vi "Set DDG External Output Enabled.vi"(8 "error in (no error)":errorcluster, 10 "uiEnabled":u32, 11 "uiIndex":u32) -> (0 "error out":errorcluster, 3 "function return":u32)   [LabVIEW 2014, in "atmcd32d.lvlib"]
doc: "unsigned int WINAPI SetDDGExternalOutputEnabled(at_u32 uiIndex, at_u32 uiEnabled);"
uses:
  atmcd32d.lvlib
  atmcd32d.dll
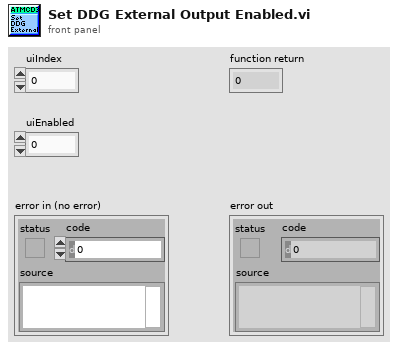
[diagram p1: front panel]
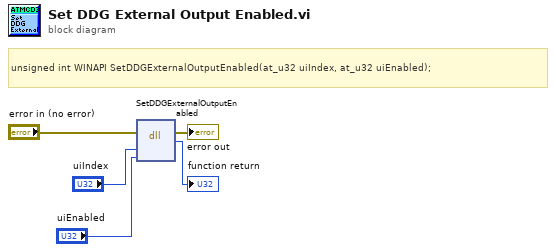
[diagram p0: block diagram]
diagram:
  # "unsigned int WINAPI SetDDGExternalOutputEnabled(at_u32 uiIndex, at_u32 uiEnabled);"
  n1 = dll-call lib="C:/Users/Bakir/Documents/Lambda2-Testing/lib/Andorlib/atmcd32d.*" fn="SetDDGExternalOutputEnabled"(error in="error in (no error)", "uiIndex"="uiIndex", "uiEnabled"="uiEnabled") -> (error out=→"error out":errorcluster, →"function return":u32)  [unwired: 4 in, 1 out]
